vi "OpenTalonDrive.vi"   [LabVIEW 2016]
uses:
  <vilib>/Rock Robotics/WPI/ThirdParty/CanMotor/TalonSRX/WPI_CANTalonSRX_APIControlMode.ctl
  <vilib>/Rock Robotics/WPI/SafetyOutput/WPI_SafetyOutputConfigMenu.ctl
  <vilib>/Rock Robotics/WPI/ThirdParty/CanMotor/TalonSRX/WPI_CANTalonSRX_APIFeedbackSelect.ctl
  <vilib>/Rock Robotics/WPI/RobotDrive/WPI_RobotDriveOpen2MotorWithExistingMotors.vi
types:
  T1 = typedef "WPI_CANTalonSRX_APIFeedbackSelect.ctl" = enum16{"Digital Quadrature Encoder", "Analog Potentiometer", "Analog Encoder", "Count on Quad-A (Rising-Edge)", "Count on Quad-A (Falling-Edge)", "CTR Magnetic Enc (Absolute)", "CTR Magnetic Enc (Relative)", "Pulse Width"}
  T2 = typedef "WPI_SafetyOutputConfigMenu.ctl" = enum16{"Enable", "Disable"}
  T3 = typedef "WPI_CANTalonSRX_APIControlMode.ctl" = enum8{"Percent VBus", "Speed", "Position", "Slave", "Unchanged / Invalid", "Voltage Compensation", "Current", "Motion Profile", "Motion Magic"}
  T4 = typedef "WPI_MotorControlDeviceRef.ctl" = cluster{"DeviceStatus":errorcluster, "Type":T5, "PWM":cluster{"PWM Channel":T6, "DeadBand":T7}, "CAN":cluster{"Device Number":u8, "SetOutput VI Ref":variant, "GetOutput VI Ref":variant, "Enable VI Ref":variant, "Disable VI Ref":variant, "Data":variant}, "Invert":bool}
  T5 = typedef "WPI_MotorControlType.ctl" = enum16{"PWM", "CAN"}
  T6 = typedef "FPGA_DIOPWMChannel.ctl" = enum8{"PWM 0", "PWM 1", "PWM 2", "PWM 3", "PWM 4", "PWM 5", "PWM 6", "PWM 7", "PWM 8", "PWM 9", "PWM MXP 0", "PWM MXP 1", "PWM MXP 2", "PWM MXP 3", "PWM MXP 4", "PWM MXP 5", "PWM MXP 6", "PWM MXP 7", "PWM MXP 8", "PWM MXP 9", "Invalid"}
  T7 = typedef "WPI_PWMDeadband.ctl" = cluster{"Name":string, "maxPositivePwm":i32, "minPositivePwm":i32, "centerPwm":i32, "maxNegativePwm":i32, "minNegativePwm":i32, "angularRange":u16}
  T8 = typedef "WPI_RobotDriveDevRef.ctl" = cluster{"DevStatus":errorcluster, "Motors[]":T4[], "Square Inputs":bool, "Max Output":dbl}
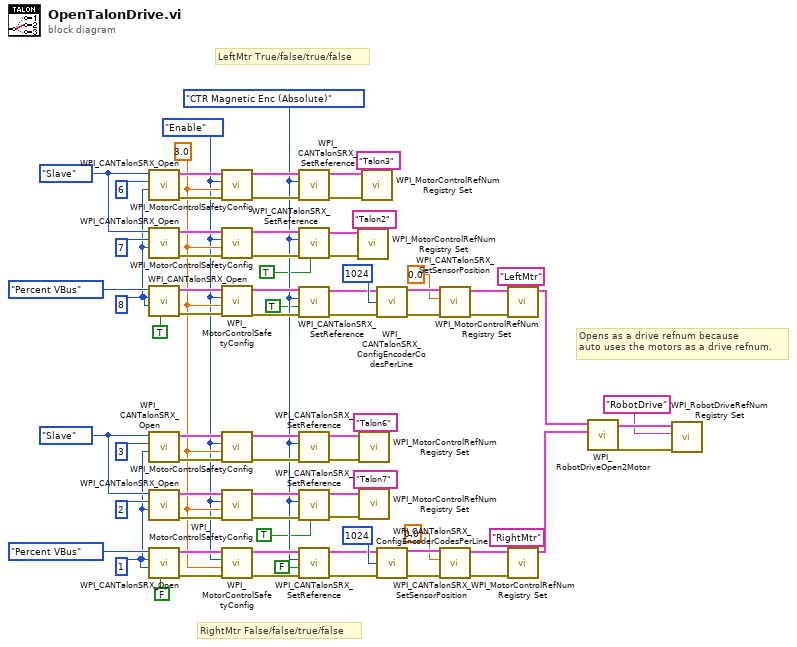
[diagram p0: block diagram]
diagram:
  w26 = WPI_CANTalonSRX_APIFeedbackSelect."CTR Magnetic Enc (Absolute)" ("Feedback Reference")
  w43 = WPI_SafetyOutputConfigMenu."Enable" ("mode")
  w11 = u8 1 ("Device Number")
  w61 = WPI_CANTalonSRX_APIControlMode."Slave" ("Control Mode")
  w44 = 3.0 ("timeout (s)")
  w10 = u8 8 ("Device Number")
  w78 = WPI_CANTalonSRX_APIControlMode."Slave" ("Control Mode")
  # "RightMtr False/false/true/false"
  # "LeftMtr True/false/true/false"
  # "Opens as a drive refnum because\nauto uses the motors as a drive refnum."
  n1 = call <vilib>:"WPI_CANTalonSRX_Open.vi"("Master Device Number"=w10, "Device Number"=u8 6, "Control Mode"=w78) -> ("error out"=w71:errorcluster, "CAN Talon SRX Ref"=w72:T4)  [unwired: 7 in]
  n2 = call <vilib>:"WPI_CANTalonSRX_Open.vi"("Master Device Number"=w10, "Device Number"=u8 7, "Control Mode"=w78) -> ("error out"=w69:errorcluster, "CAN Talon SRX Ref"=w70:T4)  [unwired: 7 in]
  n3 = call <vilib>:"WPI_CANTalonSRX_Open.vi"("Invert"=TRUE, "Master Device Number"=w10, "Device Number"=w10, "Control Mode"=WPI_CANTalonSRX_APIControlMode."Percent VBus") -> ("error out"=w73:errorcluster, "CAN Talon SRX Ref"=w74:T4)  [unwired: 6 in]
  n4 = call <vilib>:"WPI_CANTalonSRX_Open.vi"("Master Device Number"=w11, "Device Number"=u8 3, "Control Mode"=w61) -> ("error out"=w54:errorcluster, "CAN Talon SRX Ref"=w55:T4)  [unwired: 7 in]
  n5 = call <vilib>:"WPI_CANTalonSRX_Open.vi"("Master Device Number"=w11, "Device Number"=u8 2, "Control Mode"=w61) -> ("error out"=w52:errorcluster, "CAN Talon SRX Ref"=w53:T4)  [unwired: 7 in]
  n6 = call <vilib>:"WPI_CANTalonSRX_Open.vi"("Invert"=FALSE, "Master Device Number"=w11, "Device Number"=w11, "Control Mode"=WPI_CANTalonSRX_APIControlMode."Percent VBus") -> ("error out"=w56:errorcluster, "CAN Talon SRX Ref"=w57:T4)  [unwired: 6 in]
  n7 = call <vilib>:"WPI_MotorControlSafetyConfig.vi"("error in (no error)"=w71, "timeout (s)"=w44, "mode"=w43, "MotorControlDevRef"=w72) -> ("error out"=w41:errorcluster, "MotorControlDevRef"=w42:T4)  [unwired: 6 in]
  n8 = call <vilib>:"WPI_MotorControlSafetyConfig.vi"("error in (no error)"=w69, "timeout (s)"=w44, "mode"=w43, "MotorControlDevRef"=w70) -> ("error out"=w39:errorcluster, "MotorControlDevRef"=w40:T4)  [unwired: 6 in]
  n9 = call <vilib>:"WPI_MotorControlSafetyConfig.vi"("error in (no error)"=w73, "timeout (s)"=w44, "mode"=w43, "MotorControlDevRef"=w74) -> ("error out"=w29:errorcluster, "MotorControlDevRef"=w30:T4)  [unwired: 6 in]
  n10 = call <vilib>:"WPI_MotorControlSafetyConfig.vi"("error in (no error)"=w54, "timeout (s)"=w44, "mode"=w43, "MotorControlDevRef"=w55) -> ("error out"=w36:errorcluster, "MotorControlDevRef"=w35:T4)  [unwired: 6 in]
  n11 = call <vilib>:"WPI_MotorControlSafetyConfig.vi"("error in (no error)"=w52, "timeout (s)"=w44, "mode"=w43, "MotorControlDevRef"=w53) -> ("error out"=w38:errorcluster, "MotorControlDevRef"=w37:T4)  [unwired: 6 in]
  n12 = call <vilib>:"WPI_MotorControlSafetyConfig.vi"("error in (no error)"=w56, "timeout (s)"=w44, "mode"=w43, "MotorControlDevRef"=w57) -> ("error out"=w33:errorcluster, "MotorControlDevRef"=w34:T4)  [unwired: 6 in]
  n13 = call <vilib>:"WPI_CANTalonSRX_SetReference.vi"("error in (no error)"=w41, "Feedback Reference"=w26, "CAN Talon SRX Ref"=w42) -> ("error out"=w18:errorcluster, "CAN Talon SRX Ref"=w17:T4)  [unwired: 7 in]
  n14 = call <vilib>:"WPI_CANTalonSRX_SetReference.vi"("Reverse Closed-Loop Output"=TRUE, "error in (no error)"=w39, "Feedback Reference"=w26, "CAN Talon SRX Ref"=w40) -> ("error out"=w20:errorcluster, "CAN Talon SRX Ref"=w19:T4)  [unwired: 6 in]
  n15 = call <vilib>:"WPI_CANTalonSRX_SetReference.vi"("error in (no error)"=w29, "Reverse Feedback Sensor"=TRUE, "Feedback Reference"=w26, "CAN Talon SRX Ref"=w30) -> ("error out"=w27:errorcluster, "CAN Talon SRX Ref"=w28:T4)  [unwired: 6 in]
  n16 = call <vilib>:"WPI_CANTalonSRX_SetReference.vi"("error in (no error)"=w36, "Feedback Reference"=w26, "CAN Talon SRX Ref"=w35) -> ("error out"=w22:errorcluster, "CAN Talon SRX Ref"=w21:T4)  [unwired: 7 in]
  n17 = call <vilib>:"WPI_CANTalonSRX_SetReference.vi"("Reverse Closed-Loop Output"=TRUE, "error in (no error)"=w38, "Feedback Reference"=w26, "CAN Talon SRX Ref"=w37) -> ("error out"=w25:errorcluster, "CAN Talon SRX Ref"=w24:T4)  [unwired: 6 in]
  n18 = call <vilib>:"WPI_CANTalonSRX_SetReference.vi"("error in (no error)"=w33, "Reverse Feedback Sensor"=FALSE, "Feedback Reference"=w26, "CAN Talon SRX Ref"=w34) -> ("error out"=w31:errorcluster, "CAN Talon SRX Ref"=w32:T4)  [unwired: 6 in]
  n19 = call <vilib>:"WPI_MotorControlRefNum Registry Set.vi"("error in (no error)"=w20, "refnum name"="Talon2", "MotorControlDevRef"=w19) -> ()  [unwired: 7 in, 2 out]
  n20 = call <vilib>:"WPI_MotorControlRefNum Registry Set.vi"("error in (no error)"=w22, "refnum name"="Talon6", "MotorControlDevRef"=w21) -> ()  [unwired: 7 in, 2 out]
  n21 = call <vilib>:"WPI_MotorControlRefNum Registry Set.vi"("error in (no error)"=w25, "refnum name"="Talon7", "MotorControlDevRef"=w24) -> ()  [unwired: 7 in, 2 out]
  n22 = call <vilib>:"WPI_MotorControlRefNum Registry Set.vi"("error in (no error)"=w18, "refnum name"="Talon3", "MotorControlDevRef"=w17) -> ()  [unwired: 7 in, 2 out]
  n23 = call <vilib>:"WPI_CANTalonSRX_ConfigEncoderCodesPerLine.vi"("CAN Talon SRX Ref"=w28, "Number Encoder Lines\n(Counts Per Rotation)"=u32 1024 ("Number Encoder Lines\n(Counts Per Rotation)"), "error in (no error)"=w27) -> ("CAN Talon SRX Ref"=w66:T4, "error out"=w67:errorcluster)  [unwired: 11 in]
  n24 = call <vilib>:"WPI_CANTalonSRX_ConfigEncoderCodesPerLine.vi"("CAN Talon SRX Ref"=w32, "Number Encoder Lines\n(Counts Per Rotation)"=u32 1024 ("Number Encoder Lines\n(Counts Per Rotation)"), "error in (no error)"=w31) -> ("CAN Talon SRX Ref"=w49:T4, "error out"=w50:errorcluster)  [unwired: 11 in]
  n25 = call <vilib>:"WPI_CANTalonSRX_SetSensorPosition.vi"("error in (no error)"=w67, "New Sensor Position"=0.0, "CAN Talon SRX Ref"=w66) -> ("error out"=w64:errorcluster, "CAN Talon SRX Ref"=w63:T4)  [unwired: 7 in]
  n26 = call <vilib>:"WPI_CANTalonSRX_SetSensorPosition.vi"("error in (no error)"=w50, "New Sensor Position"=0.0, "CAN Talon SRX Ref"=w49) -> ("error out"=w47:errorcluster, "CAN Talon SRX Ref"=w46:T4)  [unwired: 7 in]
  n27 = call <vilib>:"WPI_MotorControlRefNum Registry Set.vi"("error in (no error)"=w64, "refnum name"="LeftMtr" ("Ref Name 1"), "MotorControlDevRef"=w63) -> ("MotorControlDevRef"=w5:T4)  [unwired: 7 in, 1 out]
  n28 = call <vilib>:"WPI_MotorControlRefNum Registry Set.vi"("error in (no error)"=w47, "refnum name"="RightMtr" ("Ref Name 2"), "MotorControlDevRef"=w46) -> ("MotorControlDevRef"=w1:T4)  [unwired: 7 in, 1 out]
  n29 = call-poly <vilib>:"WPI_RobotDriveOpen2Motor.vi"("Right Motor Dev Ref"=w1, "Left Motor Dev Ref"=w5) -> ("error out"=w3:errorcluster, "RobotDriveDevRef"=w4:T8)  [unwired: 8 in]
  n30 = call <vilib>:"WPI_RobotDriveRefNum Registry Set.vi"("error in (no error)"=w3, "refnum name"="RobotDrive", "RobotDriveDevRef"=w4) -> ()  [unwired: 7 in, 2 out]
